vi "async_home.vi"(1 "velocity":dbl, 2 "item":string(combo)="home", 3 "连接ID":refnum<k5>) -> (0 "连接ID输出":refnum<k5>)   [LabVIEW 2017]
panel:
  in  "输入簇":T1
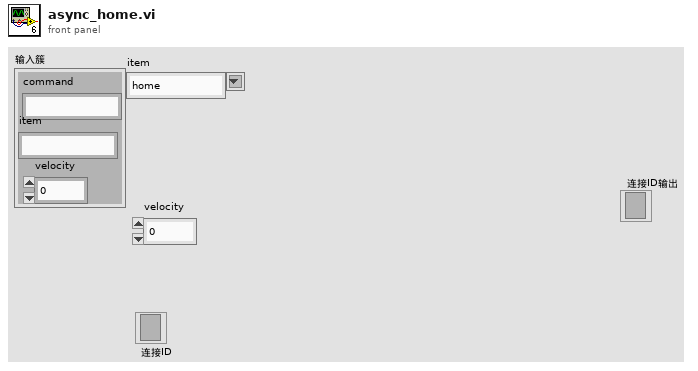
[diagram p1: front panel]
types:
  T1 = cluster{"command":string, "item":string, "velocity":dbl}
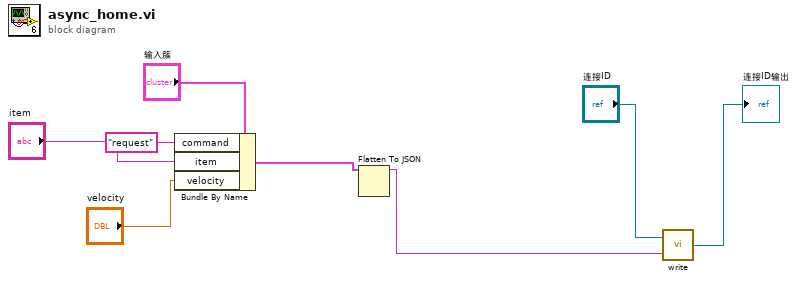
[diagram p0: block diagram]
diagram:
  n1 = Bundle By Name(cluster="输入簇", "command"="request", "item"="item", "velocity"="velocity") -> (w2:T1)
  n2 = Flatten To JSON(anything=w2) -> (JSON string=w1:string)  [unwired: 2 in, 1 out]
  n3 = call "write.vi"("数据输入"=w1, "连接ID"="连接ID") -> ("连接ID输出"=→"连接ID输出":refnum<k5>)
